vi "Write File path.vi"(8 "error in (no error)":errorcluster, 10 "File path":path, 11 "JSON in":refnum<class "JSON.lvclass">) -> (0 "error out":errorcluster, 3 "JSON out":refnum<class "JSON.lvclass">)   [LabVIEW 2018, in "JSON.lvclass"]
uses:
  JSON.lvclass
  JSON.lvclass/JSON.ctl
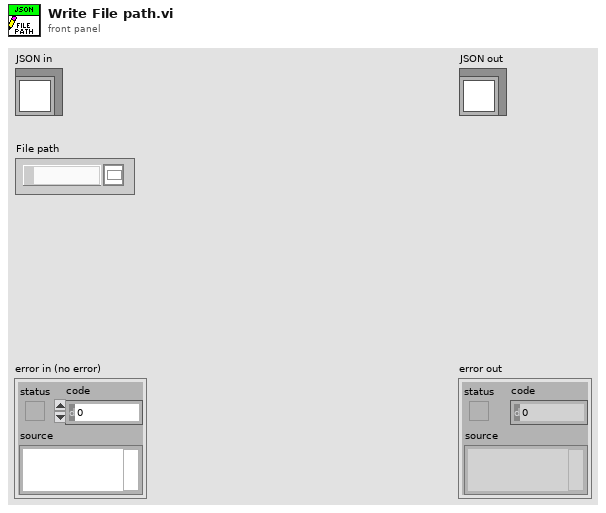
[diagram p1: front panel]
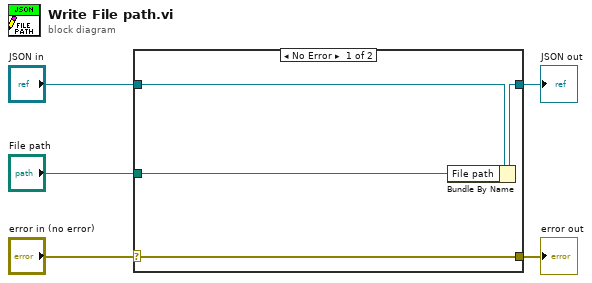
[diagram p0: block diagram]
diagram:
  n1 = case shown="No Error" "error in (no error)" {
    selector: "error in (no error)" -> [w9 w10]
    tunnel: [w9 w10] -> w4
    tunnel: [w7 w11] -> w2
    tunnel: "JSON in" -> [w8 w11]
    tunnel: "File path" -> [w6 _]
    frame No Error {
      n2 = Bundle By Name(cluster=w8, "File path"=w6) -> (w7:refnum<class "JSON.lvclass">)
    }
    frame Error {
    }
  }
  "error out" <- w4
  "JSON out" <- w2
